vi "ThermoCouple_Datafile_Append.vi"(8 "error in":errorcluster, 9 "Gradients":dbl[](array[numeric]), 10 "Temps":dbl[](array[numeric]), 11 "Path":path) -> (0 "error out":errorcluster)   [LabVIEW 2020]
uses:
  <vilib>/Utility/file.llb/Write Delimited Spreadsheet (string).vi
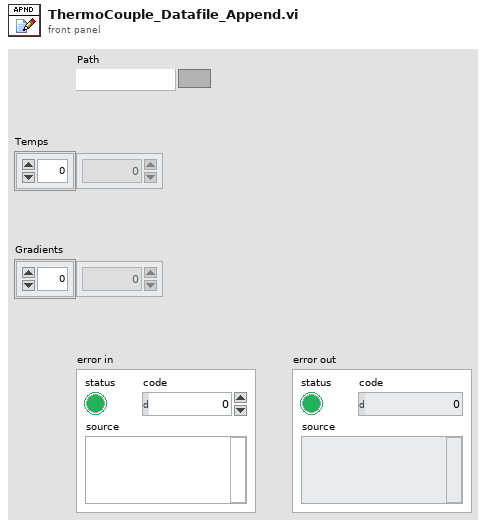
[diagram p1: front panel]
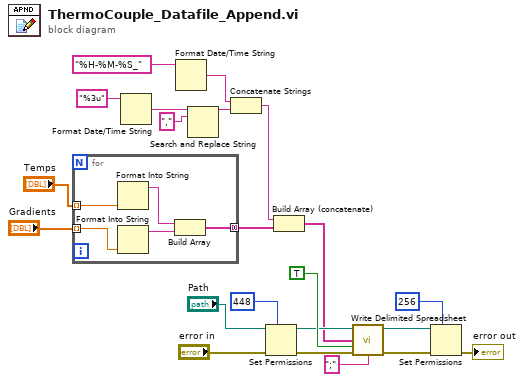
[diagram p0: block diagram]
diagram:
  n1 = for "Temp" {
    tunnel: "Temps" -> [w27] mode=indexing
    tunnel: "Gradients" -> [w26] mode=indexing
    tunnel: [w23] -> w19 mode=concatenating
    n2 = Format Into String(w27) -> (resulting string=w25:string)  [unwired: 3 in, 1 out]
    n3 = Format Into String(w26) -> (resulting string=w24:string)  [unwired: 3 in, 1 out]
    n4 = Build Array(w25, w24) -> (w23:string[])
  }
  n5 = Format Date/Time String(time format string (%c)="%3u") -> (date/time string=w6:string)  [unwired: 2 in]
  n6 = Format Date/Time String(time format string (%c)="%H-%M-%S_") -> (date/time string=w5:string)  [unwired: 2 in]
  n7 = Search and Replace String(input string=w6, search string=",") -> (result string=w7:string)  [unwired: 6 in, 3 out]
  n8 = Concatenate Strings(w5, w7) -> (w1:string)
  n9 = Set Permissions(7:i16 448 ("permissions"), 8:"error in", 11:"Path") -> (0:w11:errorcluster, 3:w16:path)  [unwired: 2 in]
  n10 = Build Array (concatenate)(w1, w19) -> (w8:string[])
  n11 = call-poly <vilib>:"Write Delimited Spreadsheet.vi"("file path (dialog if empty)"=w16, "1D data"=w8, "append to file? (new file:F)"=TRUE, "error in (no error)"=w11, "delimiter (\\t)"=";" ("delimiter (\\t)")) -> ("new file path (Not A Path if cancelled)"=w15:path, "error out"=w14:errorcluster)  [unwired: 9 in]
  n12 = Set Permissions(7:i16 256 ("permissions"), 8:w14, 11:w15) -> (0:→"error out":errorcluster)  [unwired: 2 in, 1 out]
